vi "Get Thread UI.vi"(8 "error in (no error)":errorcluster, 11 "Component UI in":refnum<class "PXImc User Interfaces.lvclass">) -> (0 "error out":errorcluster, 2 "Thread Settings UI":refnum<class "User Interface.lvclass">, 3 "Component UI out":refnum<class "PXImc User Interfaces.lvclass">)   [LabVIEW 2017, in "PXImc.lvlib" / "PXImc User Interfaces.lvclass"]
uses:
  PXImc User Interfaces.lvclass
  DSF Core.lvlibp/Classes/User Interface/User Interface.lvclass
  Thread/Thread User Interface.lvclass
  C:/Git/DSF/Components/DSF Core.lvlibp/Classes/User Interface/User Interface.lvclass
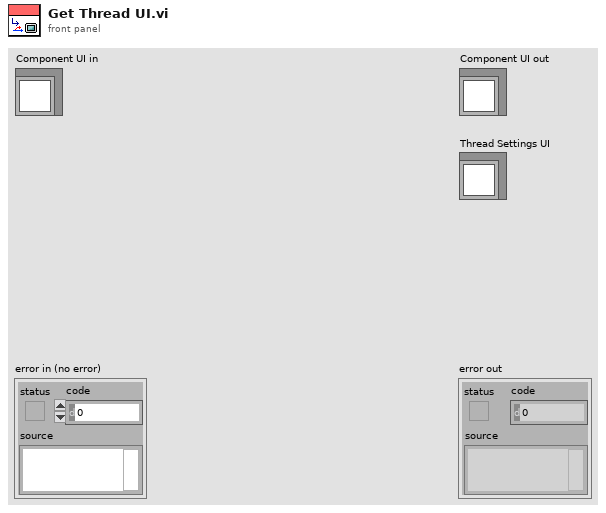
[diagram p1: front panel]
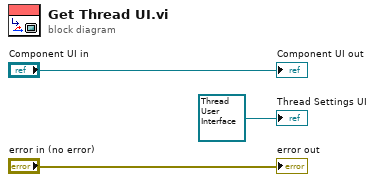
[diagram p0: block diagram]
diagram:
  "error out" <- "error in (no error)"
  "Component UI out" <- "Component UI in"
  "Thread Settings UI" <- refnum<class "Thread User Interface.lvclass"> refnum ("PXImc.lvlib:Thread User Interface.lvclass")
